vi "Load Config_Override Sections.vi"(7 "Target Folder":path, 8 "error in (no error)":errorcluster, 9 "Default File Data":T1, 10 "Default Palette Data":T2={"Display Name Override"="", "View Format"=2, "Palette Width"=0, "Help Tag"="", "Help File Path"=path "", "Palette Description"=""} {"View Format" items=["Icons", "Text", "Icons and Text"]}, 11 "Refnum in":T4) -> (0 "error out":errorcluster, 1 "File Override map":map{string, T1}(c390), 2 "Palette Override map":map{string, T2}(c390), 3 "Refnum out":T4)   [LabVIEW 2019, in "AutoMenuCreator.lvlib"]
uses:
  AutoMenuCreator.lvlib
  <vilib>/Utility/config.llb/Config Data RefNum.ctl
  Ctl/Ctl_Config_Palette Data.ctl
  <vilib>/Palette API/Palette Menu/Public Type Define/View Format.ctl
  Ctl/Ctl_Config_File Data.ctl
  <vilib>/Utility/config.llb/NI_LVConfig.lvlib
  <vilib>/Palette API/Palette Menu/Palette Menu.lvlib
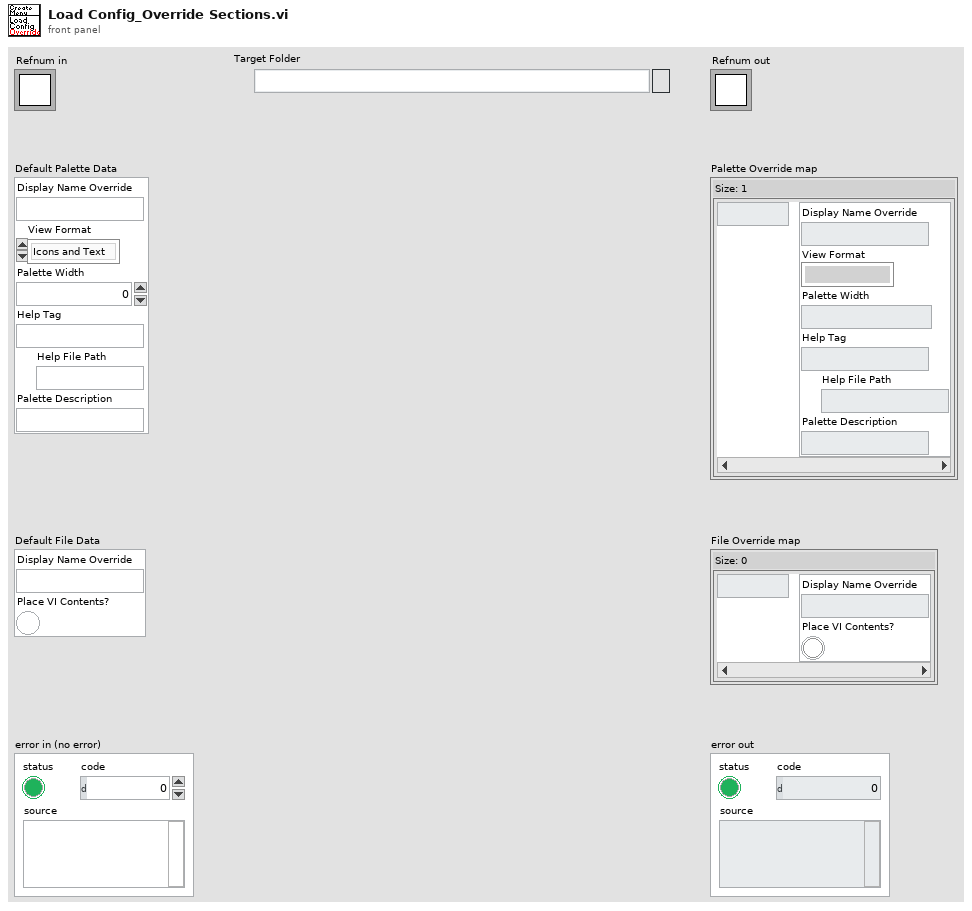
[diagram p1: front panel]
types:
  T1 = typedef "AutoMenuCreator.lvlib/Ctl_Config_File Data.ctl" = cluster{"Display Name Override":string, "Place VI Contents?":bool}
  T2 = typedef "AutoMenuCreator.lvlib/Ctl_Config_Palette Data.ctl" = cluster{"Display Name Override":string, "View Format":T3, "Palette Width":i16, "Help Tag":string, "Help File Path":path, "Palette Description":string}
  T3 = typedef "Palette Menu.lvlib/View Format.ctl" = u16
  T4 = typedef "NI_LVConfig.lvlib/Config Data RefNum.ctl" = refnum<k1>
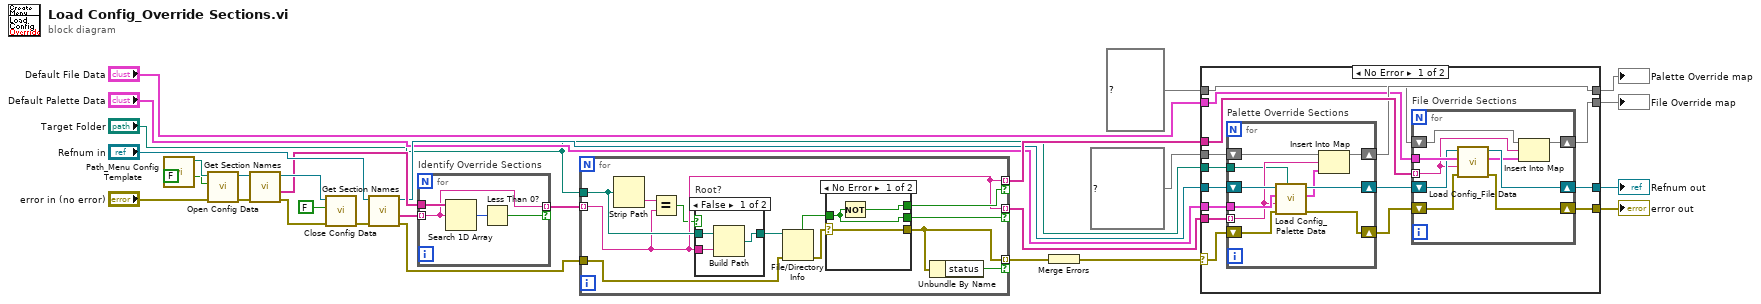
[diagram p0: block diagram]
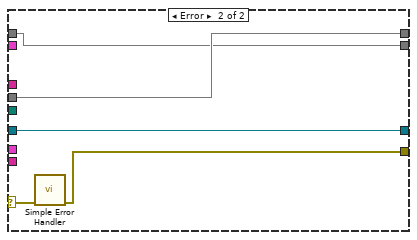
[diagram p2: hidden frame]
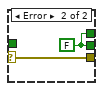
[diagram p4: hidden frame]
diagram:
  n1 = call "Path_Menu Config Template.vi"() -> ("Menu Config Template path"=w26:path)  [unwired: 11 in]
  n2 = call <vilib>:"Open Config Data.vi"("error in (no error)"="error in (no error)", "create file if necessary (T)"=FALSE, "configuration file path"=w26) -> ("error out"=w23:errorcluster, "refnum"=w24:T4)  [unwired: 6 in, 1 out]
  n3 = call <vilib>:"Get Section Names.vi"("error in (no error)"=w23, "refnum"=w24) -> ("error out"=w20:errorcluster, "section names"=w18:string[], "refnum out"=w21:T4)  [unwired: 7 in]
  n4 = call <vilib>:"Close Config Data.vi"("error in (no error)"=w20, "write file if changed (T)"=FALSE, "refnum"=w21) -> ("error out"=w17:errorcluster)  [unwired: 7 in, 1 out]
  n5 = call <vilib>:"Get Section Names.vi"("error in (no error)"=w17, "refnum"="Refnum in") -> ("error out"=w15:errorcluster, "section names"=w27:string[], "refnum out"=w8:T4)  [unwired: 7 in]
  n6 = for "Identify Override Sections" {
    tunnel: w27 -> [w30] mode=indexing
    tunnel: w18 -> [w31]
    tunnel: [w30] -> w16 mode=indexing if=w29
    n7 = Search 1D Array(1D array=w31, element=w30) -> (index of element=w32:i32)  [unwired: 1 in]
    n8 = Less Than 0?(x=w32) -> (x < 0?=w29:bool)
  }
  n9 = for {
    tunnel: w16 -> [w34] mode=indexing
    tunnel: "Target Folder" -> [w36]
    tunnel: w15 -> [w43]
    tunnel: [w41] -> w14 mode=indexing if=w40
    tunnel: [w34] -> w12 mode=indexing if=w38
    tunnel: [w34] -> w13 mode=indexing if=w37
    n10 = Strip Path(path=w36) -> (name=w35:string)  [unwired: 1 out]
    n11 = Equal?(x=w35, y=w34) -> (x = y?=w33:bool)
    n12 = case "Root?" shown="False" w33 {
      tunnel: [w47 w48] -> w44
      tunnel: w36 -> [w46 w48]
      tunnel: w34 -> [w45 _]
      frame False {
        n13 = Build Path(base path=w46, name or relative path=w45) -> (appended path=w47:path)
      }
      frame True {
      }
    }
    n14 = File/Directory Info(path=w44, error in=w43) -> (directory=w39:bool, error out=w42:errorcluster)  [unwired: 5 out]
    n15 = case shown="No Error" w42 {
      selector: w42 -> [w49 w53]
      tunnel: [w49 w53] -> w41
      tunnel: w39 -> [w50 _]
      tunnel: [w51 w52] -> w38
      tunnel: [w50 w52] -> w37
      frame No Error {
        n16 = Not(x=w50) -> (.not. x?=w51:bool)
      }
      frame Error {
        w52 = FALSE
      }
    }
    n17 = Unbundle By Name(w41) -> ("status"=w40:bool)
  }
  n18 = Merge Errors(w14) -> (w11:errorcluster)
  n19 = case shown="No Error" w11 {
    selector: w11 -> [w65 w92]
    tunnel: w13 -> [w68 _]
    tunnel: w12 -> [w67 _]
    tunnel: "Default Palette Data" -> [w66 _]
    tunnel: [w60 w91] -> w10
    tunnel: "Default File Data" -> [w56 _]
    tunnel: w8 -> [w64 w90]
    tunnel: [w61 w90] -> w7
    tunnel: map{string, T2} {} ("map") -> [w59 w89]
    tunnel: "Target Folder" -> [w58 _]
    tunnel: [w57 w89] -> w3
    tunnel: [w55 w88] -> w1
    tunnel: map{string, T1} {} ("map") -> [w54 w88]
    frame No Error {
      n20 = for "Palette Override Sections" {
        tunnel: w68 -> [w79] mode=indexing
        tunnel: w66 -> [w87]
        shift-right: [w85] -> w62
        shift-left: w65 -> [w86]
        shift-right: [w83] -> w63
        shift-left: w64 -> [w84]
        shift-right: [w81] -> w57
        shift-left: w59 -> [w82]
        tunnel: w58 -> [w78]
        n21 = call "Load Config_Palette Data.vi"("Target Folder"=w78, "error in (no error)"=w86, "Section (\"Default Palette Data\")"=w79, "Palette Data in"=w87, "Refnum in"=w84) -> ("error out"=w85:errorcluster, "Palette Data out"=w80:T2, "Refnum out"=w83:T4)  [unwired: 4 in]
        n22 = Insert Into Map(map in=w82, key=w79, value=w80) -> (map out=w81:map{string, T2})  [unwired: 2 out]
      }
      n23 = for "File Override Sections" {
        tunnel: w67 -> [w69] mode=indexing
        tunnel: w56 -> [w77]
        shift-right: [w73] -> w60
        shift-left: w62 -> [w75]
        shift-right: [w74] -> w61
        shift-left: w63 -> [w76]
        shift-right: [w71] -> w55
        shift-left: w54 -> [w72]
        n24 = call "Load Config_File Data.vi"("error in (no error)"=w75, "Section (\"Default File Data\")"=w69, "File Data in"=w77, "Refnum in"=w76) -> ("error out"=w73:errorcluster, "File Data out"=w70:T1, "Refnum out"=w74:T4)  [unwired: 5 in]
        n25 = Insert Into Map(map in=w72, key=w69, value=w70) -> (map out=w71:map{string, T1})  [unwired: 2 out]
      }
    }
    frame Error {
      n26 = call <vilib>:"Simple Error Handler.vi"("error in (no error)"=w92) -> ("error out"=w91:errorcluster)  [unwired: 4 in, 4 out]
    }
  }
  "error out" <- w10
  "Refnum out" <- w7
  "Palette Override map" <- w3
  "File Override map" <- w1
